vi "Read Micron Optics Digitizer Configuration.vi"(8 "error in (no error)":errorcluster, 11 "Micron Optics Driver in":refnum<class "Micron Optics Driver.lvclass">) -> (0 "error out":errorcluster, 2 "Micron Optics Digitizer Configuration":T1={"Post-trigger delay"=0.01, "Post-trigger duration"=0.1, "Rate"=1000000.0, "Ranges"=[10.0], "Re-name channels"=[], "Active channels"="0:1", "External\nclock"=FALSE, "Reference channel"=-1, "Detection Setting IDs"=[130, 130], "Stream and average"=FALSE, "Address"="10.0.0.55"} {"Rate" format="%#_8pHz"; "Post-trigger duration" format="%#_6ps"; "Post-trigger delay" format="%#_6ps"; "Ranges" format="%#_6pV"}, 3 "Micron Optics Driver out":refnum<class "Micron Optics Driver.lvclass">)   [LabVIEW 2024, in "Micron Optics Driver.lvclass"]
uses:
  Micron Optics Driver.lvclass
  Micron Optics Driver.lvclass/Micron Optics Driver.ctl
  Micron optics didgitizer configuration.ctl
panel:
  # "Pulse config"
  # "Monitor config"
  # "CH1\n.\n.\n.\n.\n.\nCH4"
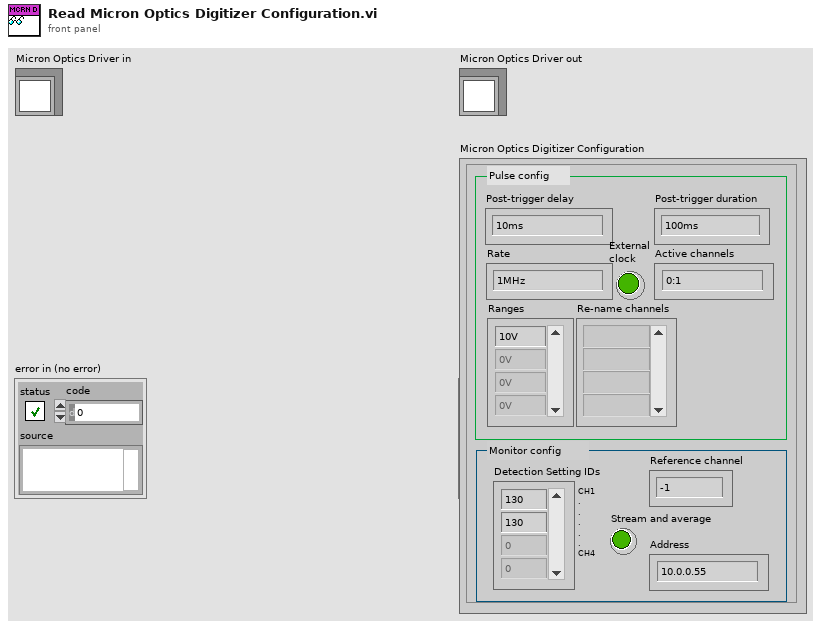
[diagram p1: front panel]
types:
  T1 = typedef "Micron optics didgitizer configuration.ctl" = cluster{"Post-trigger delay":dbl, "Post-trigger duration":dbl, "Rate":dbl, "Ranges":dbl[], "Re-name channels":string[], "Active channels":string, "External\nclock":bool, "Reference channel":i32, "Detection Setting IDs":u8[], "Stream and average":bool, "Address":string}
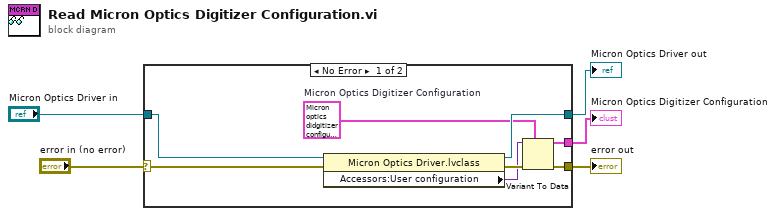
[diagram p0: block diagram]
diagram:
  n1 = case shown="No Error" "error in (no error)" {
    selector: "error in (no error)" -> [w13 w14]
    tunnel: [w9 w14] -> w4
    tunnel: [w11 w15] -> w2
    tunnel: "Micron Optics Driver in" -> [w12 w15]
    tunnel: [w6 _] -> w1
    frame No Error {
      w8 = T1 {"Post-trigger delay"=0.01, "Post-trigger duration"=0.1, "Rate"=1000000.0, "Ranges"=[10.0], "Re-name channels"=[], "Active channels"="0:1", "External\nclock"=FALSE, "Reference channel"=-1, "Detection Setting IDs"=[130, 130], "Stream and average"=FALSE, "Address"="10.0.0.55"}  # Micron Optics Digitizer Configuration
      n2 = property class="Micron Optics Driver.lvclass"(reference=w12, error in=w13) -> (reference out=w11:refnum<class "Micron Optics Driver.lvclass">, error out=w10:errorcluster, "Accessors:User configuration"=w7:variant)
      n3 = Variant To Data(error in=w10, type=w8, Variant=w7) -> (data=w6:T1, error out=w9:errorcluster)
    }
    frame Error {
    }
  }
  "error out" <- w4
  "Micron Optics Driver out" <- w2
  "Micron Optics Digitizer Configuration" <- w1
